vi "2D Real FFT.vi"(1 "X":dbl[][](array[numeric]) format="%.2f") -> (0 "FFT {X}":cdb[][](array[numeric]) format="%.2f")   [LabVIEW 2024]
uses:
  <vilib>/Analysis/2dsp.llb/Real FFT.vi
  <vilib>/Analysis/2dsp.llb/Complex FFT.vi
  <vilib>/Analysis/NI_AALPro.lvlib
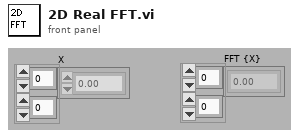
[diagram p1: front panel]
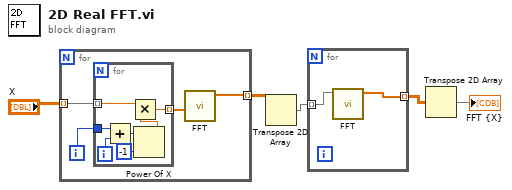
[diagram p0: block diagram]
diagram:
  n1 = for {
    tunnel: "X" -> [w7] mode=indexing
    tunnel: [w9] -> w4 mode=indexing
    i -> [w8]
    n2 = for {
      tunnel: w8 -> [w15]
      tunnel: w7 -> [w11] mode=indexing
      tunnel: [w10] -> w6 mode=indexing
      i -> [w16]
      n3 = Add(x=w15, y=w16) -> (x+y=w14:i32)
      n4 = Power Of X(1:-1, 2:w14) -> (0:w12:dbl)
      n5 = Multiply(x=w11, y=w12) -> (x*y=w10:dbl)
    }
    n6 = call-poly <vilib>:"FFT.vi"("X"=w6) -> ("FFT {X}"=w9:cdb[])  [unwired: 9 in, 1 out]
  }
  n7 = Transpose 2D Array(2D array=w4) -> (transposed array=w5:cdb[][])
  n8 = for {
    tunnel: w5 -> [w18] mode=indexing
    tunnel: [w17] -> w2 mode=indexing
    n9 = call-poly <vilib>:"FFT.vi"("X"=w18) -> ("FFT {X}"=w17:cdb[])  [unwired: 9 in, 1 out]
  }
  n10 = Transpose 2D Array(2D array=w2) -> (transposed array=→"FFT {X}":cdb[][])
